vi "Get Default Platano AppData Folder.vi"() -> (0 "error out":errorcluster, 2 "Platano AppData":path)   [LabVIEW 2021, in "Bananas.lvlib" / "Platano.lvclass"]
uses:
  Platano.lvclass
  <vilib>/Utility/sysdir.llb/System Directory Type.ctl
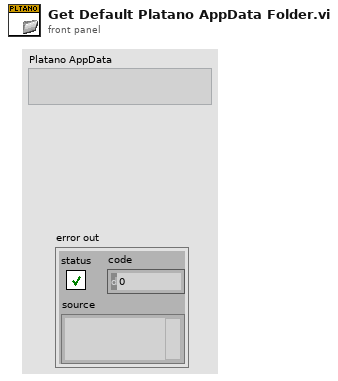
[diagram p1: front panel]
types:
  T1 = typedef "System Directory Type.ctl" = i32
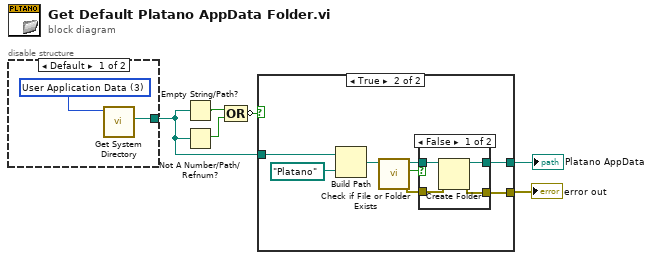
[diagram p0: block diagram]
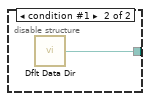
[diagram p2: hidden frame]
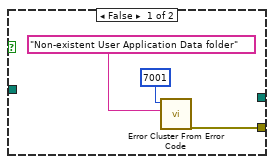
[diagram p3: hidden frame]
diagram:
  n1 = disable-structure shown="Default" {
    disable-tunnel: [w8 w9] -> w2
    frame condition #0 (active) {
      w7 = T1 3 items=["User Home"=0, "User Desktop"=1, "User Documents"=2, "User Application Data"=3, "User Preferences"=4, "User Temporary"=5, "Public Documents"=6, "Public Application Data"=7, "Public Preferences"=8, "Public Cache"=13, "System Core Libraries"=9, "System Installed Libraries"=10, "Application Files"=11, "Boot Volume Root"=12] ("system directory type")
      n2 = call <vilib>:"Get System Directory.vi"("system directory type"=w7) -> ("system directory"=w8:path)  [unwired: 10 in]
    }
    frame condition #1 {
      n3 = call <vilib>:"Dflt Data Dir.vi"() -> ("App:Default Data Directory"=w9:path)
    }
  }
  n4 = Empty String/Path?(string/path=w2) -> (empty?=w3:bool)
  n5 = Not A Number/Path/Refnum?(number/path/refnum=w2) -> (NaN/Path/Refnum?=w4:bool)
  n6 = Compound Arithmetic op=OR(w3, w4) -> (invert w1:bool)
  n7 = case shown="True" w1 {
    tunnel: w2 -> [_ w19]
    tunnel: [_ w14] -> w5
    tunnel: [w12 w13] -> w6
    frame False {
      n8 = call <vilib>:"Error Cluster From Error Code.vi"("error message (\"\")"="Non-existent User Application Data folder" ("error message (\"\")"), "error code (0)"=7001) -> ("error out"=w12:errorcluster)  [unwired: 7 in]
    }
    frame True {
      n9 = Build Path(base path=w19, name or relative path=path "Platano") -> (appended path=w18:path)
      n10 = call <vilib>:"Check if File or Folder Exists.vi"("path"=w18) -> ("error out"=w16:errorcluster, "file or folder exists?"=w15:bool, "dup path"=w17:path)  [unwired: 8 in]
      n11 = case shown="False" w15 {
        tunnel: [w24 w26] -> w14
        tunnel: w17 -> [w23 w26]
        tunnel: w16 -> [w22 w25]
        tunnel: [w21 w25] -> w13
        frame False {
          n12 = Create Folder(path (use dialog)=w23, error in=w22) -> (created path=w24:path, error out=w21:errorcluster)  [unwired: 1 in, 1 out]
        }
        frame True {
        }
      }
    }
  }
  "error out" <- w6
  "Platano AppData" <- w5
